vi "Stop Core.vi"(10 "final error code":i32, 11 "uService Template in":refnum<class "Common GUI v3.lvclass">) -> (3 "uService Template out":refnum<class "Common GUI v3.lvclass">)   [LabVIEW 2026, in "TALOS.lvlib" / "Common GUI v3.lvlib" / "Common GUI v3.lvclass"]
doc: "(<B>Filename</B>: Actor Framework.lvlib:Actor.lvclass:Stop Core.vi)\n\nDefines what the actor does before it stops. Use the <B>final error code</B> input to determine whether the actor shut down in response to an error.\n\nBy default, this method passes the Stop message along to all auto-stop nested actors. A descendant class may override this method to define additional behavior, such as shutting down any processes the actor initiated in its override of the Actor Core method."
uses:
  Common GUI v3.lvclass
  Father of all uServices/Father of all uServices/Father of all uServices.lvclass
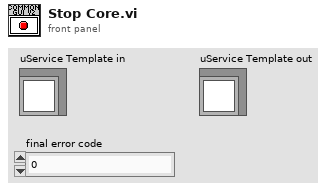
[diagram p1: front panel]
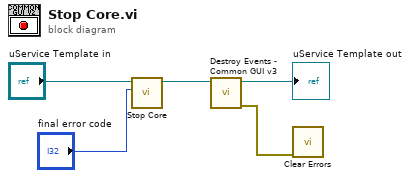
[diagram p0: block diagram]
diagram:
  n1 = call-parent "Stop Core.vi"("final error code"="final error code", "uService Template in"="uService Template in") -> ("uService Template out"=w3:refnum<class "Common GUI v3.lvclass">)  [unwired: 9 in]
  n2 = call "Destroy Events - Common GUI v3.vi"("Common GUI uService in"=w3) -> ("error out"=w1:errorcluster, "Common GUI uService out"=→"uService Template out":refnum<class "Common GUI v3.lvclass">)  [unwired: 9 in]
  n3 = call <vilib>:"Clear Errors.vi"("error in (no error)"=w1) -> ()  [unwired: 5 in, 2 out]
